vi "GlobalRecParam7.vi"(1 "New Parameter Index":u32, 2 "New Parameter Value":sgl, 3 "Function select":string) -> (0 "1D Output Array":sgl[](array[numeric]))   [LabVIEW 2015]
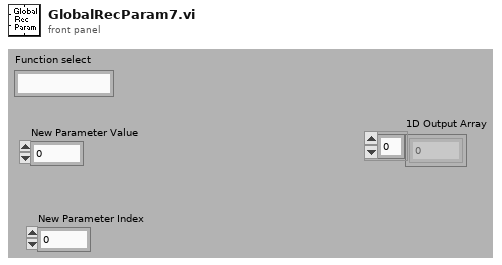
[diagram p1: front panel]
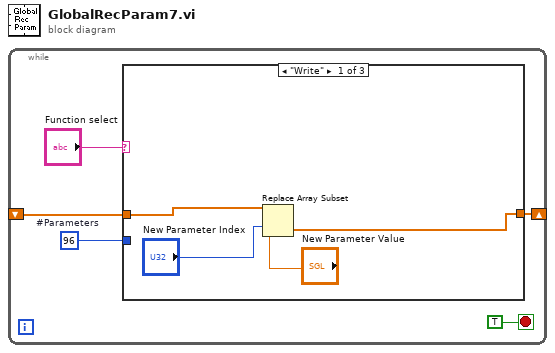
[diagram p0: block diagram]
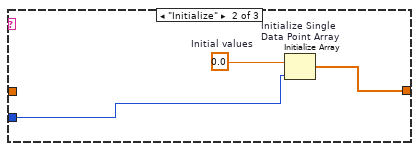
[diagram p2: hidden frame]
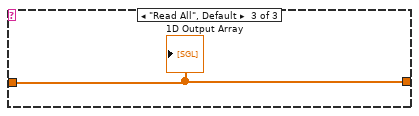
[diagram p3: hidden frame]
diagram:
  n1 = while {
    shift-right: [w2] -> _
    shift-left: _ -> [w1]
    stop <- TRUE stop-if-true
    w3 = 96  # #Parameters
    n2 = case shown="\"Write\"" "Function select" {
      tunnel: w3 -> [_ w12 _]
      tunnel: [w9 w10 w13] -> w2
      tunnel: w1 -> [w8 _ w13]
      frame "Write" {
        n3 = Replace Array Subset(array=w8, new element="New Parameter Value", index="New Parameter Index") -> (w9:sgl[])
      }
      frame "Initialize" {
        w11 = sgl 0.0  # Initial values
        n4 = Initialize Array "Initialize Single\nData Point Array"(w11, w12) -> (w10:sgl[])
      }
      frame "Read All", Default {
        "1D Output Array" <- w13
      }
    }
  }
